vi "Create Side View SCM Spark Scene.vi"(2 "error in (no error)":errorcluster, 3 "Spark Coordinates (cm, rad, cm)":cluster{"r":sgl, "theta":sgl, "z":sgl}[](array[cluster])) -> (0 "error out":errorcluster, 1 "reference out":refnum<vi>)   [LabVIEW 2013, in "Breakdown Acoustics Controls.lvlib"]
uses:
  <vilib>/Utility/miscctls.llb/LV3DPointTypeDef.ctl
  <vilib>/picture/3D Picture Control/Object/Create Object (name).vi
  Breakdown Acoustics Controls.lvlib
  <vilib>/picture/3D Picture Control/NI_3D Picture Control.lvlib
panel:
  out "Cavity Length (u)":sgl=1.2
  out "Cavity Radius (u)":sgl=1.2
  out "Graphical Units per Meter":dbl
  out "Cavity Side View":refnum<vi>(3d-picture)
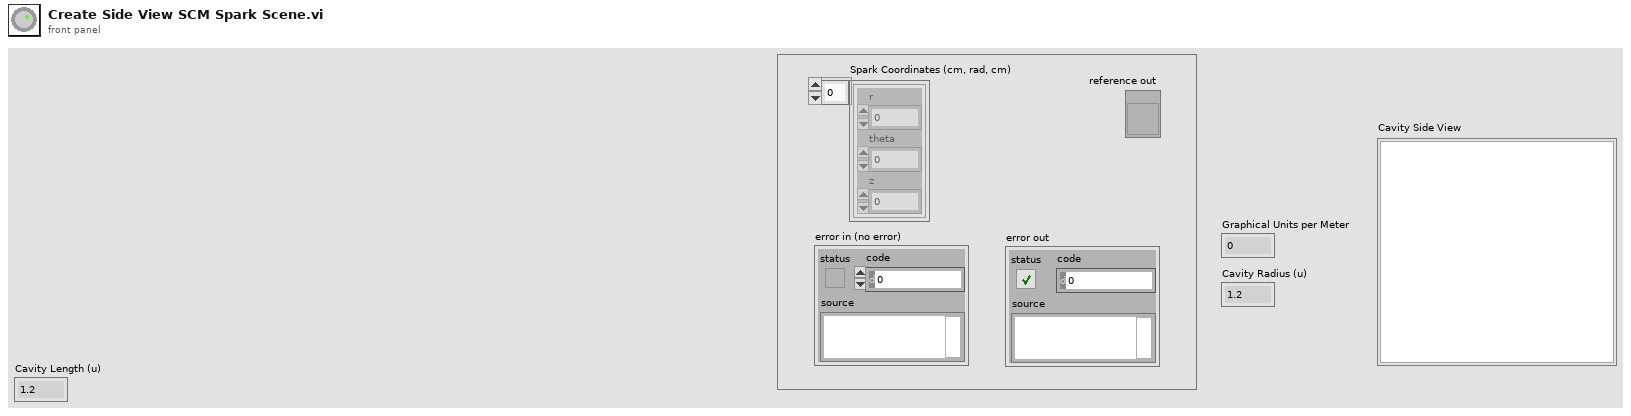
[diagram p1: front panel]
types:
  T1 = cluster{"Red":sgl, "Green":sgl, "Blue":sgl, "Alpha":sgl}[]
  T2 = typedef "LV3DPointTypeDef.ctl" = cluster{"X":sgl, "Y":sgl, "Z":sgl}
  T3 = cluster{"Red":sgl, "Green":sgl, "Blue":sgl, "Alpha":sgl}
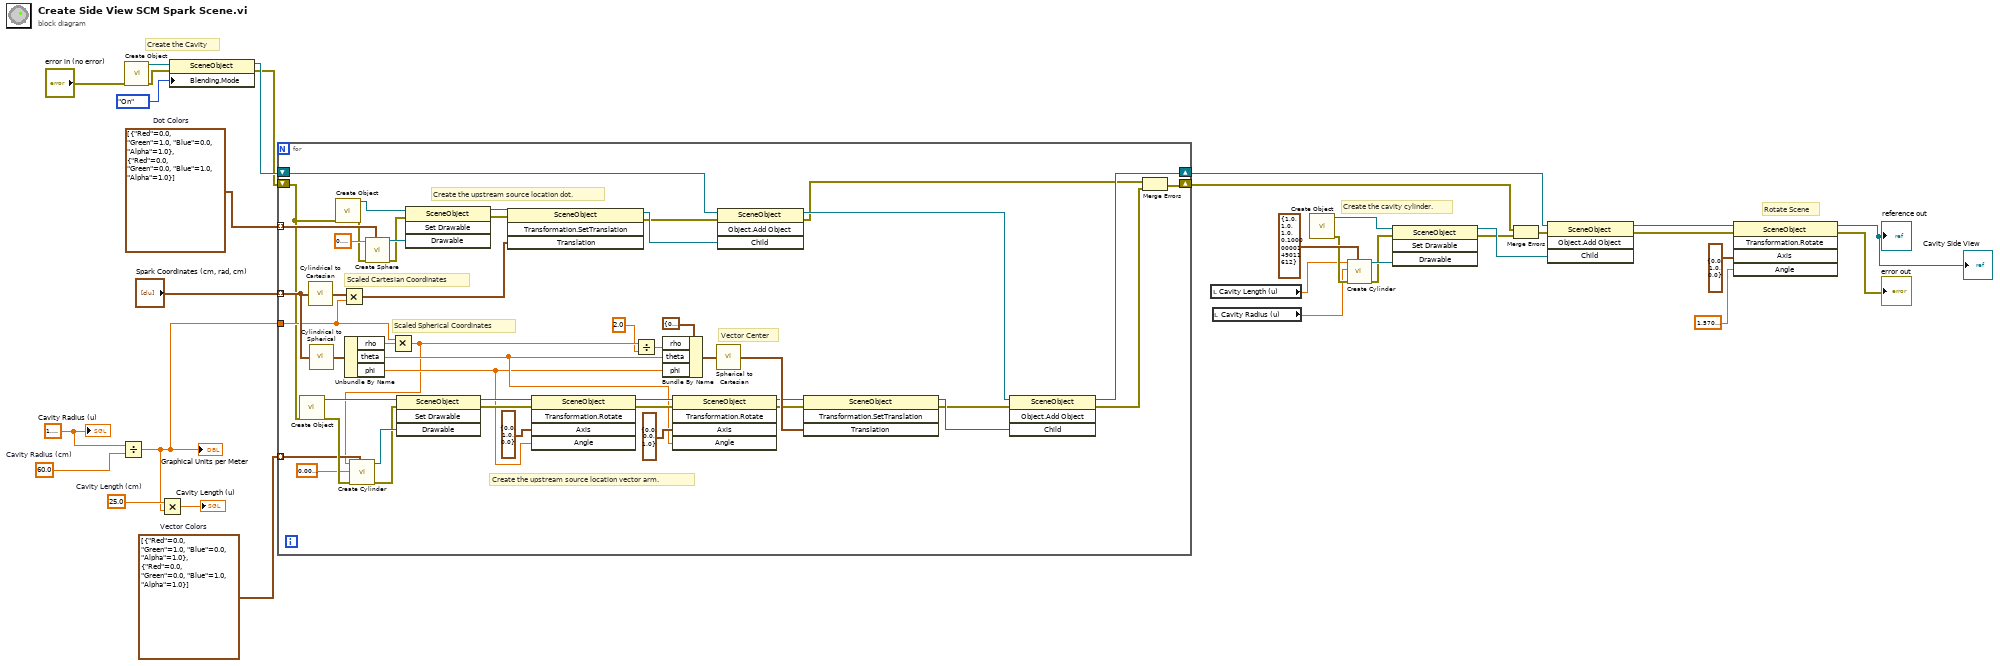
[diagram p0: block diagram]
diagram:
  w6 = T1 [{"Red"=0.0, "Green"=1.0, "Blue"=0.0, "Alpha"=1.0}, {"Red"=0.0, "Green"=0.0, "Blue"=1.0, "Alpha"=1.0}]  # Dot Colors
  w5 = T1 [{"Red"=0.0, "Green"=1.0, "Blue"=0.0, "Alpha"=1.0}, {"Red"=0.0, "Green"=0.0, "Blue"=1.0, "Alpha"=1.0}]  # Vector Colors
  w13 = sgl 25.0  # Cavity Length (cm)
  w25 = 60.0  # Cavity Radius (cm)
  w23 = sgl 1.2 ("Cavity Radius (u)")
  # "Create the Cavity"
  # "Rotate Scene"
  # "Create the cavity cylinder."
  n1 = Divide ("graphical units per meter")(x=w23, y=w25) -> (x/y=w7:dbl)
  "Graphical Units per Meter" <- w7
  n2 = call-poly <vilib>:"Create Object.vi"("error in (no error)"="error in (no error)") -> ("error out"=w29:errorcluster, "Scene:New Object"=w30:refnum<vi>)  [unwired: 9 in]
  n3 = Multiply(x=w13, y=w7) -> (x*y=→"Cavity Length (u)":dbl)
  n4 = property class="SceneObject"(reference=w30, error in=w29, "Blending.Mode"=enum16{"Inherit Value", "Off", "On"}."On" ("Blending:Mode")) -> (reference out=w2:refnum<vi>, error out=w1:errorcluster)
  n5 = for {
    tunnel: "Spark Coordinates (cm, rad, cm)" -> [w77] mode=indexing
    tunnel: w7 -> [w50]
    tunnel: w6 -> [w71] mode=indexing
    tunnel: w5 -> [w49] mode=indexing
    shift-right: [w43] -> w4
    shift-left: w2 -> [w42]
    shift-right: [w37] -> w3
    shift-left: w1 -> [w39]
    # "Vector Center"
    # "Create the upstream source location vector arm."
    # "Create the upstream source location dot."
    # "Scaled Cartesian Coordinates"
    # "Scaled Spherical Coordinates"
    n6 = call-poly <vilib>:"Create Object.vi"("error in (no error)"=w39) -> ("error out"=w54:errorcluster, "Scene:New Object"=w52:refnum<vi>)  [unwired: 9 in]
    n7 = call "Cylindrical to Cartesian.vi"("Cylindrical\nCoordinates"=w77) -> ("Cartesian\nCoordinates"=w78:cluster{"x":dbl, "y":dbl, "z":dbl})  [unwired: 4 in]
    n8 = call "Cylindrical to Spherical.vi"("Cylindrical\nCoordinates"=w77) -> ("Spherical\nCoordinates"=w79:cluster{"rho":dbl, "theta":dbl, "phi":dbl})  [unwired: 4 in]
    n9 = call-poly <vilib>:"Create Object.vi"("error in (no error)"=w39) -> ("error out"=w70:errorcluster, "Scene:New Object"=w74:refnum<vi>)  [unwired: 9 in]
    n10 = Multiply(x=w78, y=w50) -> (x*y=w69:cluster{"x":dbl, "y":dbl, "z":dbl})
    n11 = Unbundle By Name(w79) -> ("rho"=w51:dbl, "theta"=w48:dbl, "phi"=w47:dbl)
    n12 = call <vilib>:"Create Sphere.vi"("Color"=w71, "error in (no error)"=w70, "Radius"=sgl 0.1) -> ("error out"=w41:errorcluster, "New Sphere Refnum"=w73:refnum<vi>)  [unwired: 7 in]
    n13 = Multiply(x=w50, y=w51) -> (x*y=w34:dbl)
    n14 = call <vilib>:"Create Cylinder.vi"("Color"=w49, "error in (no error)"=w54, "Radius"=sgl 0.01, "Height"=w34) -> ("error out"=w55:errorcluster, "New Cylinder Refnum"=w62:refnum<vi>)  [unwired: 6 in]
    n15 = invoke class="SceneObject" method="Set Drawable"(reference=w52, error in=w55, "Drawable"=w62) -> (reference out=w63:refnum<vi>, error out=w64:errorcluster)  [unwired: 1 in, 2 out]
    n16 = invoke class="SceneObject" method="Set Drawable"(reference=w74, error in=w41, "Drawable"=w73) -> (reference out=w75:refnum<vi>, error out=w76:errorcluster)  [unwired: 1 in, 2 out]
    n17 = invoke class="SceneObject" method="Transformation.SetTranslation"(reference=w75, error in=w76, "Translation"=w69) -> (reference out=w46:refnum<vi>, error out=w40:errorcluster)  [unwired: 1 in, 2 out]
    n18 = invoke class="SceneObject" method="Transformation.Rotate"(reference=w63, error in=w64, "Axis"=T2 {"X"=0.0, "Y"=1.0, "Z"=0.0}, "Angle"=w47) -> (reference out=w58:refnum<vi>, error out=w59:errorcluster)  [unwired: 1 in, 3 out]
    n19 = Divide(x=w34, y=2.0) -> (x/y=w65:dbl)
    n20 = Bundle By Name(cluster=cluster{"rho":dbl, "theta":dbl, "phi":dbl} {"rho"=0.0, "theta"=0.0, "phi"=0.0} ("Spherical\nCoordinates"), "rho"=w65, "theta"=w48, "phi"=w47) -> (w66:cluster{"rho":dbl, "theta":dbl, "phi":dbl})
    n21 = invoke class="SceneObject" method="Transformation.Rotate"(reference=w58, error in=w59, "Axis"=T2 {"X"=0.0, "Y"=0.0, "Z"=1.0}, "Angle"=w48) -> (reference out=w60:refnum<vi>, error out=w61:errorcluster)  [unwired: 1 in, 3 out]
    n22 = call "Spherical to Cartesian.vi"("Spherical\nCoordinates"=w66) -> ("Cartesian\nCoordinates"=w68:cluster{"x":dbl, "y":dbl, "z":dbl})  [unwired: 4 in]
    n23 = invoke class="SceneObject" method="Object.Add Object"(reference=w42, error in=w40, "Child"=w46) -> (reference out=w44:refnum<vi>, error out=w35:errorcluster)  [unwired: 1 in, 2 out]
    n24 = invoke class="SceneObject" method="Transformation.SetTranslation"(reference=w60, error in=w61, "Translation"=w68) -> (reference out=w45:refnum<vi>, error out=w38:errorcluster)  [unwired: 1 in, 2 out]
    n25 = invoke class="SceneObject" method="Object.Add Object"(reference=w44, error in=w38, "Child"=w45) -> (reference out=w43:refnum<vi>, error out=w36:errorcluster)  [unwired: 1 in, 2 out]
    n26 = Merge Errors(w35, w36) -> (w37:errorcluster)
  }
  n27 = local read "Cavity Length (u)"() -> (w11:sgl)
  n28 = local read "Cavity Radius (u)"() -> (w10:sgl)
  n29 = call-poly <vilib>:"Create Object.vi"() -> ("error out"=w22:errorcluster, "Scene:New Object"=w27:refnum<vi>)  [unwired: 10 in]
  n30 = call <vilib>:"Create Cylinder.vi"("Color"=T3 {"Red"=1.0, "Green"=1.0, "Blue"=1.0, "Alpha"=0.1}, "error in (no error)"=w22, "Radius"=w10, "Height"=w11) -> ("error out"=w21:errorcluster, "New Cylinder Refnum"=w31:refnum<vi>)  [unwired: 6 in]
  n31 = invoke class="SceneObject" method="Set Drawable"(reference=w27, error in=w21, "Drawable"=w31) -> (reference out=w26:refnum<vi>, error out=w20:errorcluster)  [unwired: 1 in, 2 out]
  n32 = Merge Errors(w3, w20) -> (w24:errorcluster)
  n33 = invoke class="SceneObject" method="Object.Add Object"(reference=w4, error in=w24, "Child"=w26) -> (reference out=w15:refnum<vi>, error out=w14:errorcluster)  [unwired: 1 in, 2 out]
  n34 = invoke class="SceneObject" method="Transformation.Rotate"(reference=w15, error in=w14, "Axis"=T2 {"X"=0.0, "Y"=1.0, "Z"=0.0}, "Angle"=sgl 1.571) -> (reference out=→"reference out" →"Cavity Side View":refnum<vi>, error out=→"error out":errorcluster)  [unwired: 1 in, 3 out]
  "Cavity Radius (u)" <- w23
